vi "Stop Event.vi"() -> (3 "Stop event":refnum<user-event>)   [LabVIEW 2020, in "RxnRover.lvlib"]
doc: "Effectively provides a singleton \"Stop\" event instance. The event instance is created on the first call and returned on all subsequent calls."
uses:
  RxnRover.lvlib
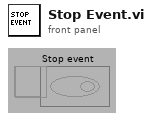
[diagram p1: front panel]
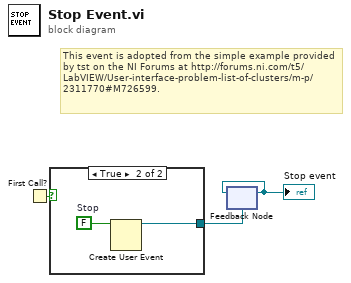
[diagram p0: block diagram]
diagram:
  # "This event is adopted from the simple example provided by tst on the NI Forums at http://forums.ni.com/t5/LabVIEW/User-interface-problem-list-of-clusters/m-p/2311770#M726599."
  n1 = First Call?() -> (First Call?: T/F=w2:bool)
  n2 = case shown="True" w2 {
    tunnel: [_ w5] -> w3
    frame False {
    }
    frame True {
      w4 = FALSE  # Stop
      n3 = Create User Event(user event datatype=w4) -> (user event=w5:refnum<user-event>)  [unwired: 1 in, 1 out]
    }
  }
  n4 = feedback #1(w3) -> (w1:refnum<user-event>)
  "Stop event" <- w1
  n5 = feedback-in #1(w1) -> ()
